vi "FTW-XML-Destroy.vi"(0 "XML Node":refnum<k20>, 11 "error in":errorcluster) -> (15 "error out":errorcluster)   [LabVIEW 2015]
panel:
  # "Inputs"
  # "Outputs"
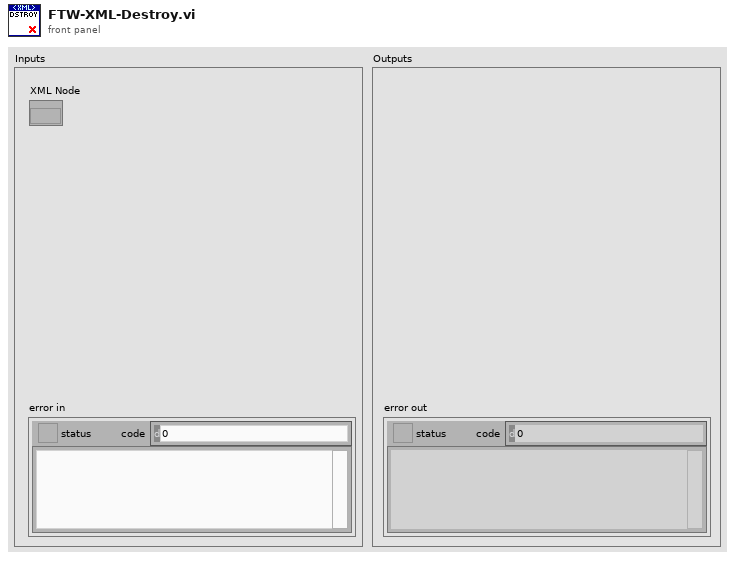
[diagram p1: front panel]
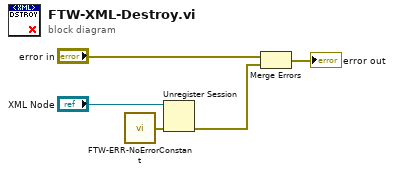
[diagram p0: block diagram]
diagram:
  n1 = call "FTW-ERR-NoErrorConstant.vi"() -> ("no error"=w1:errorcluster)
  n2 = Unregister Session(8:w1, 11:"XML Node") -> (0:w2:errorcluster)
  n3 = Merge Errors("error in", w2) -> (→"error out":errorcluster)
